vi "TCP Client_32.vi"(0 "CMD":i32, 1 "remote port \nor service name":u16, 2 "ID_Trace":i32, 3 "error in (no error)":errorcluster, 4 "timeout ms":i32, 5 "Address":string, 8 "TRACE_SIZE":i32) -> (6 "Output cluster":T1, 7 "R_message 1":string, 10 "error out":errorcluster)   [LabVIEW 2022 SP3]
uses:
  <vilib>/Utility/error.llb/Error Cluster From Error Code.vi
  <vilib>/ErrorRing/Error Ring.xnode
panel:
  out "R_Data string length":cluster{i32}
  out "W_Data string length: \nbytes written 2":i32
  out "W_Data string_flat":string
  # "0-> OCP_IF_CMD_TRACE_READ = 0, //LV: SIZE - CMD - ID || RESPONSE: SIZE - DATA\n1->\tOCP_IF_CMD_TRACE_RESET, //SIZE - CMD - ID || RESPONSE: SIZE\n2-> OCP_IF_CMD_TRACE_GET_SIZE, //SIZE - CMD - ID || RESPONSE: SIZE - TRACE_SIZE (4 bztes)\n3->\tOCP_IF_CMD_TRACE_SET_SIZE, //SIZE - CMD - ID - TRACE_SIZE ( 4 bytes) || RESPONSE: SIZE\n4->\tOCP_IF_CMD_TRACE_GET_NUMBER_SIGNALS, //SIZE - CMD - ID || RESPONSE: SIZE - NB_SIGNALS (4 bytes)\n5->\tOCP_IF_CMD_TRACE_GET_SIGNALS_NAMES, //SIZE - CMD - ID || RESPONSE: SIZE - string\n6->\tOCP_IF_CMD_TRACE_GET_NUMBER_TRACES, //SIZE - CMD  || RESPONSE: SIZE - NB_TRACES (4 bytes)\n7->\tOCP_IF_CMD_TRACE_GET_TRACES_NAMES, //SIZE - CMD || RESPONSE: SIZE - string"
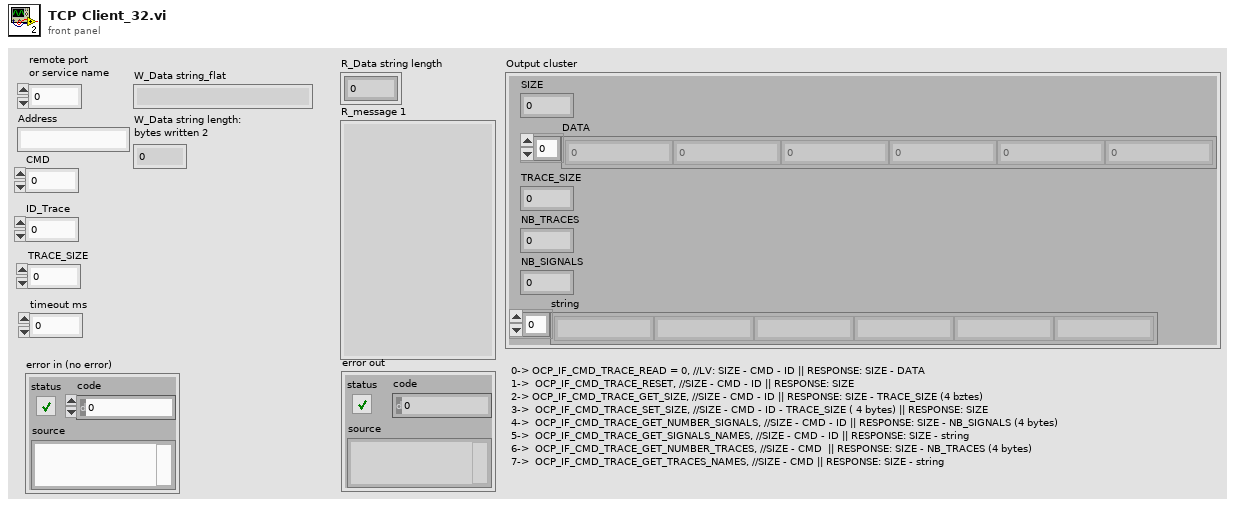
[diagram p1: front panel]
types:
  T1 = cluster{"SIZE":i32, "DATA":sgl[], "TRACE_SIZE":i32, "NB_TRACES":i32, "NB_SIGNALS":i32, "string":string[]}
  T2 = enum16{"big-endian, network order", "native, host order", "little-endian"}
  T3 = enum16{"Standard", "Buffered", "CRLF", "Immediate"}
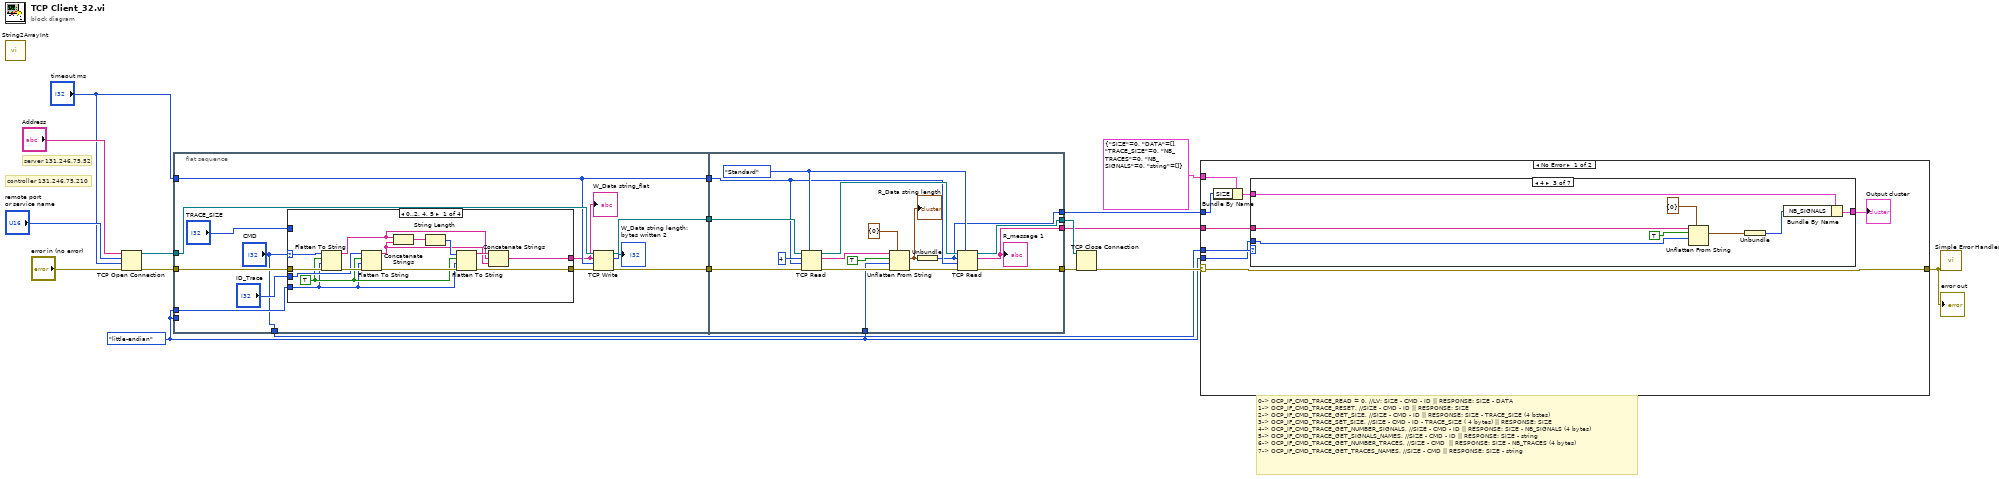
[diagram p0: block diagram]
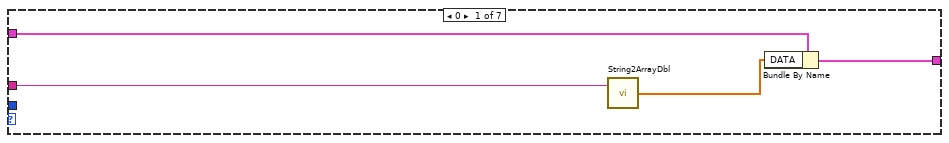
[diagram p2: hidden frame]
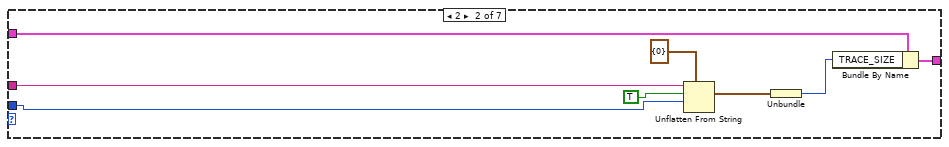
[diagram p3: hidden frame]
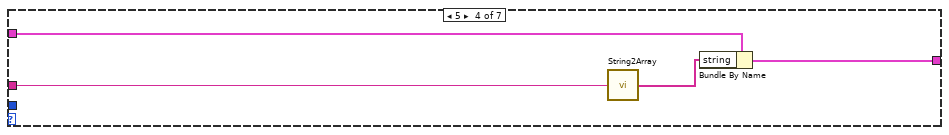
[diagram p4: hidden frame]
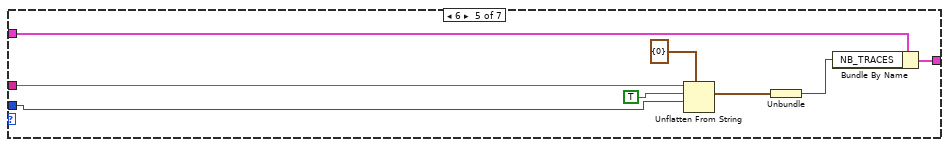
[diagram p5: hidden frame]
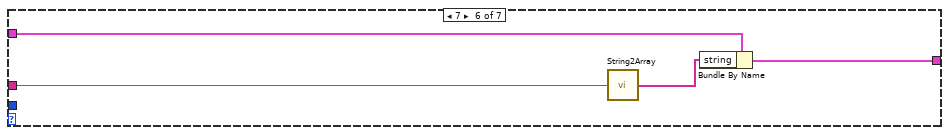
[diagram p6: hidden frame]
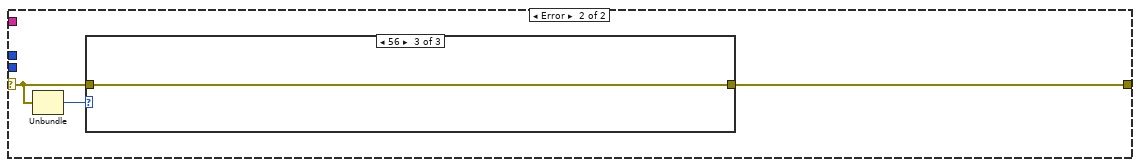
[diagram p8: hidden frame]
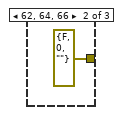
[diagram p10: hidden frame]
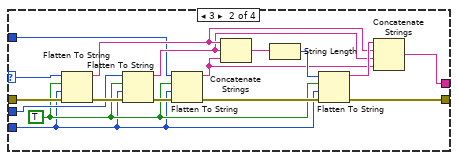
[diagram p11: hidden frame]
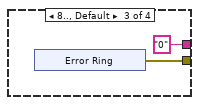
[diagram p12: hidden frame]
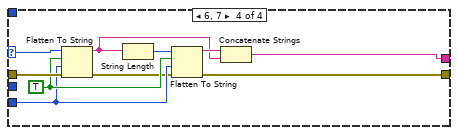
[diagram p13: hidden frame]
diagram:
  w2 = T2."little-endian" ("byte order (0:big-endian, network order)")
  # "0-> OCP_IF_CMD_TRACE_READ = 0, //LV: SIZE - CMD - ID || RESPONSE: SIZE - DATA\n1->\tOCP_IF_CMD_TRACE_RESET, //SIZE - CMD - ID || RESPONSE: SIZE\n2-> OCP_IF_CMD_TRACE_GET_SIZE, //SIZE - CMD - ID || RESPONSE: SIZE - TRACE_SIZE (4 bztes)\n3->\tOCP_IF_CMD_TRACE_SET_SIZE, //SIZE - CMD - ID - TRACE_SIZE ( 4 bytes) || RESPONSE: SIZE\n4->\tOCP_IF_CMD_TRACE_GET_NUMBER_SIGNALS, //SIZE - CMD - ID || RESPONSE: SIZE - NB_SIGNALS (4 bytes)\n5->\tOCP_IF_CMD_TRACE_GET_SIGNALS_NAMES, //SIZE - CMD - ID || RESPONSE: SIZE - string\n6->\tOCP_IF_CMD_TRACE_GET_NUMBER_TRACES, //SIZE - CMD  || RESPONSE: SIZE - NB_TRACES (4 bytes)\n7->\tOCP_IF_CMD_TRACE_GET_TRACES_NAMES, //SIZE - CMD || RESPONSE: SIZE - string"
  # "controller 131.246.75.210"
  # "server 131.246.75.52"
  n1 = call "String2ArrayInt.vi"() -> ()  [unwired: 2 in, 2 out]
  n2 = TCP Open Connection(address="Address", remote port or service name="remote port \nor service name", timeout ms (60000)="timeout ms", error in (no error)="error in (no error)") -> (connection ID=w16:refnum<k5>, error out=w15:errorcluster)  [unwired: 1 in]
  n3 = flat-sequence {
    tunnel: w16 -> [w29]
    tunnel: w15 -> [w25]
    tunnel: [w28] -> w14
    tunnel: [w27] -> w13
    tunnel: w2 -> [_]
    tunnel: "timeout ms" -> [w26]
    tunnel: [w26] -> w6
    tunnel: w2 -> [w24]
    tunnel: ["CMD"] -> w5
    tunnel: w14 -> [w93]
    tunnel: w13 -> [w92]
    tunnel: [w91] -> w10
    tunnel: [w90] -> w9
    tunnel: w2 -> [w83]
    tunnel: w6 -> [w81]
    tunnel: [w80] -> w4
    tunnel: [w79] -> w1
    frame #0 {
      n4 = case shown="0..2, 4, 5" "CMD" {
        selector: "CMD" -> [w42 w59 _ w77]
        tunnel: w25 -> [w44 w61 _ w78]
        tunnel: w24 -> [w35 w47 _ w73]
        tunnel: "ID_Trace" -> [w41 w58 _ _]
        tunnel: [w34 w54 "0" w72] -> w23
        tunnel: [w33 w46 w63 w70] -> w22
        tunnel: "TRACE_SIZE" -> [_ w49 _ _]
        frame 0..2, 4, 5 {
          w36 = TRUE ("prepend array or string size? (T)")
          n5 = Flatten To String(anything=w42, prepend array or string size? (T)=w36, byte order (0:big-endian, network order)=w35, error in (no error)=w44) -> (data string=w32:string, error out=w43:errorcluster)  [unwired: 1 out]
          n6 = Flatten To String(anything=w41, prepend array or string size? (T)=w36, byte order (0:big-endian, network order)=w35, error in (no error)=w43) -> (data string=w31:string, error out=w38:errorcluster)  [unwired: 1 out]
          n7 = Concatenate Strings(w32, w31) -> (w40:string)
          n8 = String Length(string=w40) -> (length=w39:i32)
          n9 = Flatten To String(anything=w39, prepend array or string size? (T)=w36, byte order (0:big-endian, network order)=w35, error in (no error)=w38) -> (data string=w37:string, error out=w33:errorcluster)  [unwired: 1 out]
          n10 = Concatenate Strings(w37, w32, w31) -> (w34:string)
        }
        frame 3 {
          w48 = TRUE ("prepend array or string size? (T)")
          n11 = Flatten To String(anything=w59, prepend array or string size? (T)=w48, byte order (0:big-endian, network order)=w47, error in (no error)=w61) -> (data string=w53:string, error out=w60:errorcluster)  [unwired: 1 out]
          n12 = Flatten To String(anything=w58, prepend array or string size? (T)=w48, byte order (0:big-endian, network order)=w47, error in (no error)=w60) -> (data string=w52:string, error out=w51:errorcluster)  [unwired: 1 out]
          n13 = Flatten To String(anything=w49, prepend array or string size? (T)=w48, byte order (0:big-endian, network order)=w47, error in (no error)=w51) -> (data string=w45:string, error out=w50:errorcluster)  [unwired: 1 out]
          n14 = Concatenate Strings(w53, w52, w45) -> (w57:string)
          n15 = String Length(string=w57) -> (length=w56:i32)
          n16 = Flatten To String(anything=w56, prepend array or string size? (T)=w48, byte order (0:big-endian, network order)=w47, error in (no error)=w50) -> (data string=w55:string, error out=w46:errorcluster)  [unwired: 1 out]
          n17 = Concatenate Strings(w55, w53, w52, w45) -> (w54:string)
        }
        frame 8.., Default {
          n18 = xnode "Error Ring"() -> ("error out"=w63:errorcluster)
        }
        frame 6, 7 {
          w74 = TRUE ("prepend array or string size? (T)")
          n19 = Flatten To String(anything=w77, prepend array or string size? (T)=w74, byte order (0:big-endian, network order)=w73, error in (no error)=w78) -> (data string=w69:string, error out=w71:errorcluster)  [unwired: 1 out]
          n20 = String Length(string=w69) -> (length=w76:i32)
          n21 = Flatten To String(anything=w76, prepend array or string size? (T)=w74, byte order (0:big-endian, network order)=w73, error in (no error)=w71) -> (data string=w75:string, error out=w70:errorcluster)  [unwired: 1 out]
          n22 = Concatenate Strings(w75, w69) -> (w72:string)
        }
      }
      "W_Data string_flat" <- w23
      n23 = TCP Write(connection ID=w29, data in=w23, error in (no error)=w22, 9:w26) -> (connection ID out=w27:refnum<k5>, bytes written=→"W_Data string length: \nbytes written 2":i32, error out=w28:errorcluster)
    }
    frame #1 {
      w95 = T3."Standard" ("mode (standard)")
      n24 = TCP Read(connection ID=w92, bytes to read=4, error in (no error)=w93, 7:w95, 9:w81) -> (connection ID out=w94:refnum<k5>, data out=w89:string, error out=w85:errorcluster)
      n25 = Unflatten From String(type=cluster{i32} {0}, binary string=w89, data includes array or string size? (T)=TRUE, byte order (0:big-endian, network order)=w83, error in (no error)=w85) -> (value=w86:cluster{i32}, error out=w84:errorcluster)  [unwired: 1 out]
      "R_Data string length" <- w86
      n26 = Unbundle(w86) -> (w79:i32)
      n27 = TCP Read(connection ID=w94, bytes to read=w79, error in (no error)=w84, 7:w95, 9:w81) -> (connection ID out=w91:refnum<k5>, data out=w80:string, error out=w90:errorcluster)
      "R_message 1" <- w80
    }
  }
  n28 = TCP Close Connection(connection ID=w10, error in (no error)=w9) -> (error out=w11:errorcluster)  [unwired: 1 in, 1 out]
  n29 = case shown="No Error" w11 {
    selector: w11 -> [w103 w142]
    tunnel: [w103 w141] -> w12
    tunnel: w5 -> [w102 _]
    tunnel: w4 -> [w98 _]
    tunnel: T1 {"SIZE"=0, "DATA"=[], "TRACE_SIZE"=0, "NB_TRACES"=0, "NB_SIGNALS"=0, "string"=[]} ("input cluster") -> [w101 _]
    tunnel: w2 -> [w96 _]
    tunnel: w1 -> [w99 _]
    frame No Error {
      n30 = Bundle By Name(cluster=w101, "SIZE"=w99) -> (w100:T1)
      n31 = case shown="4" w102 {
        tunnel: [w106 w114 w122 w126 w135 w138 w140] -> w97
        tunnel: w100 -> [w107 w115 w123 w127 w132 w139 w140]
        tunnel: w98 -> [w104 w112 w119 w125 w130 w137 _]
        tunnel: w96 -> [_ w110 w118 _ w131 _ _]
        frame 0 {
          n32 = call "String2ArrayDbl.vi"("R_message 1"=w104) -> ("Array"=w105:sgl[])  [unwired: 1 in]
          n33 = Bundle By Name(cluster=w107, "DATA"=w105) -> (w106:T1)
        }
        frame 2 {
          n34 = Unflatten From String(type=cluster{i32} {0}, binary string=w112, data includes array or string size? (T)=TRUE, byte order (0:big-endian, network order)=w110) -> (value=w109:cluster{i32})  [unwired: 1 in, 2 out]
          n35 = Unbundle(w109) -> (w108:i32)
          n36 = Bundle By Name(cluster=w115, "TRACE_SIZE"=w108) -> (w114:T1)
        }
        frame 4 {
          n37 = Unflatten From String(type=cluster{i32} {0}, binary string=w119, data includes array or string size? (T)=TRUE, byte order (0:big-endian, network order)=w118) -> (value=w120:cluster{i32})  [unwired: 1 in, 2 out]
          n38 = Unbundle(w120) -> (w116:i32)
          n39 = Bundle By Name(cluster=w123, "NB_SIGNALS"=w116) -> (w122:T1)
        }
        frame 5 {
          n40 = call "String2Array.vi"("R_message 1"=w125) -> ("Array 2"=w124:string[])
          n41 = Bundle By Name(cluster=w127, "string"=w124) -> (w126:T1)
        }
        frame 6 {
          n42 = Unflatten From String(type=cluster{i32} {0}, binary string=w130, data includes array or string size? (T)=TRUE, byte order (0:big-endian, network order)=w131) -> (value=w134:cluster{i32})  [unwired: 1 in, 2 out]
          n43 = Unbundle(w134) -> (w128:i32)
          n44 = Bundle By Name(cluster=w132, "NB_TRACES"=w128) -> (w135:T1)
        }
        frame 7 {
          n45 = call "String2Array.vi"("R_message 1"=w137) -> ("Array 2"=w136:string[])
          n46 = Bundle By Name(cluster=w139, "string"=w136) -> (w138:T1)
        }
        frame 8.., Default {
        }
      }
      "Output cluster" <- w97
    }
    frame Error {
      n47 = Unbundle(w142) -> ("code"=w143:i32)  [unwired: 2 out]
      n48 = case shown="56" w143 {
        tunnel: [w144 errorcluster {"status"=FALSE, "code"=0, "source"=""} ("error IO") w146] -> w141
        tunnel: w142 -> [w144 _ w146]
        frame 0, Default {
        }
        frame 62, 64, 66 {
        }
        frame 56 {
        }
      }
    }
  }
  "error out" <- w12
  n49 = call <vilib>:"Simple Error Handler.vi"("error in (no error)"=w12) -> ()  [unwired: 4 in, 5 out]
